vi "MAVLink Heartbeat.vi"(7 "FGV Method":T2, 11 "HeartBeat in":T1 {"custom_mode" format="%x"}) -> (3 "HeartBeat out":T1 {"custom_mode" format="%x"})   [LabVIEW 2014]
uses:
  MAVLink/Controls/MAVLink Heartbeat.ctl
  Controls/FGV Methods.ctl
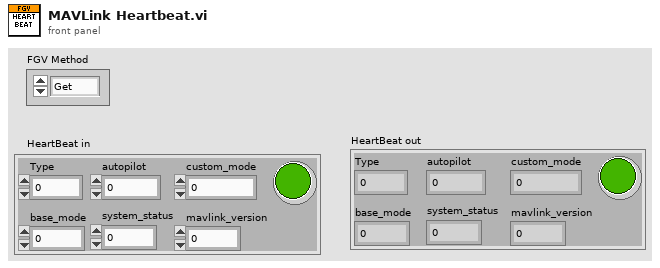
[diagram p1: front panel]
types:
  T1 = typedef "MAVLink Heartbeat.ctl" = cluster{"custom_mode":u32, "Type":u8, "autopilot":u8, "base_mode":u8, "system_status":u8, "mavlink_version":u8, "heartbeat":bool}
  T2 = typedef "FGV Methods.ctl" = enum16{"Get", "Set"}
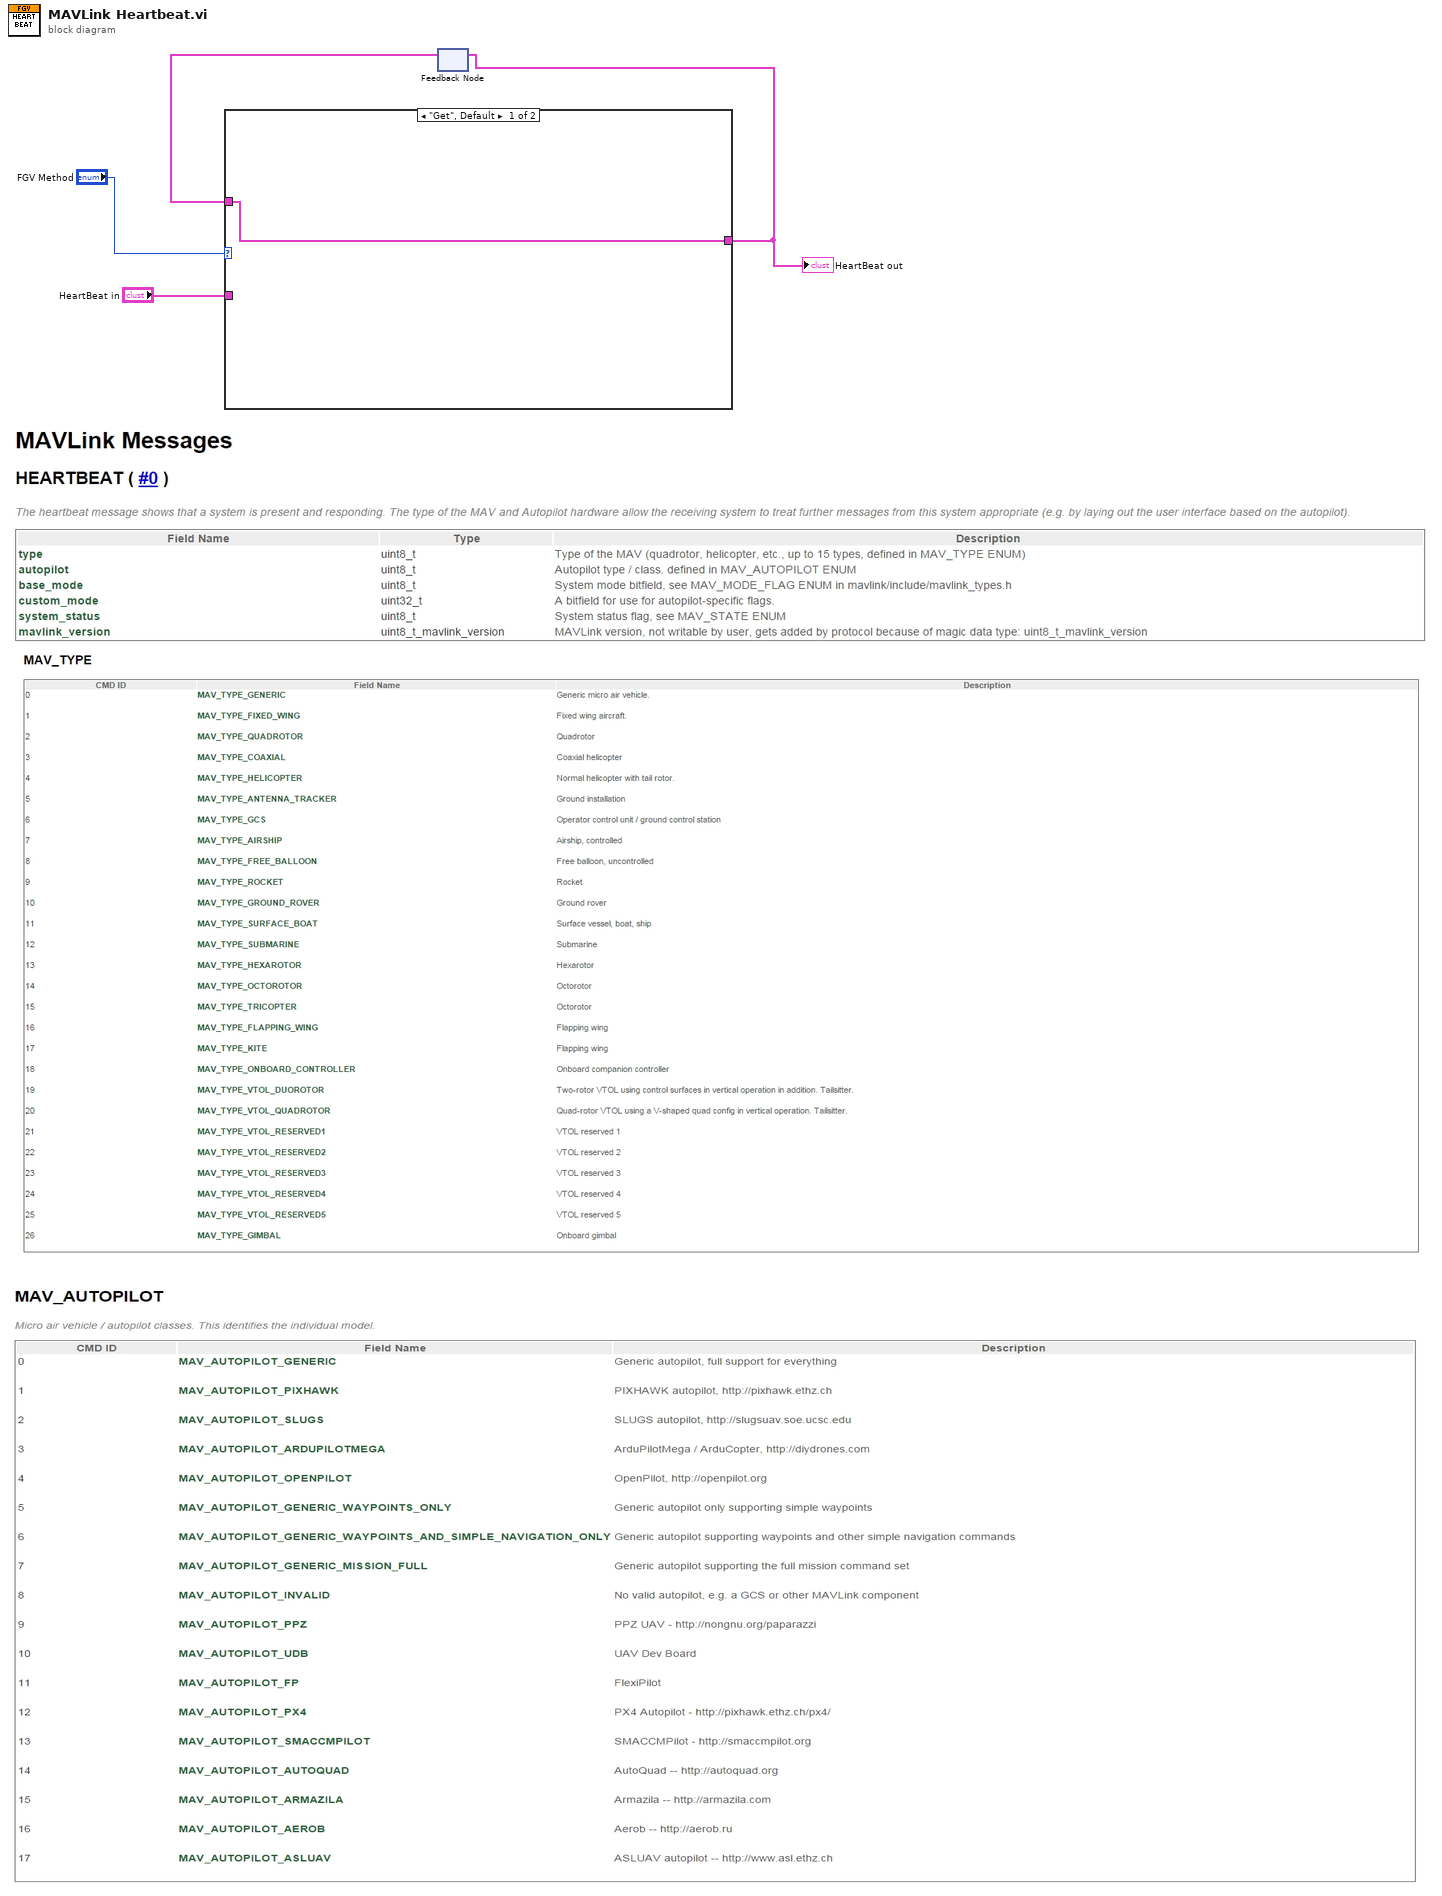
[diagram p0: block diagram]
diagram:
  n1 = feedback #1() -> (w1:T1)  [unwired: 1 in]
  n2 = case shown="\"Get\", Default" "FGV Method" {
    tunnel: "HeartBeat in" -> [_ w6]
    tunnel: [w5 w6] -> w2
    tunnel: w1 -> [w5 _]
    frame "Get", Default {
    }
    frame "Set" {
    }
  }
  "HeartBeat out" <- w2
  n3 = feedback-in #1(w2) -> ()
